vi "Init.vi"(8 "error in (no error)":errorcluster, 11 "Data in":refnum<class "Blackboard_Boolean.lvclass">) -> (0 "error out":errorcluster, 3 "Data out":refnum<class "Blackboard_Boolean.lvclass">)   [LabVIEW 2021, in "Blackboard_Boolean.lvclass"]
doc: "Abstract Data Classes 2.1.1.12\nTim Streeter - TSA\nCopyright (c) 2024, TSA"
uses:
  Blackboard_Boolean.lvclass
  Blackboard_Boolean.lvclass/Blackboard_Boolean.ctl
  Blackboard.lvclass
  <vilib>/TSA/Abstract Data Classes/Abs_Types/Type/Abs_Type.lvclass
  <vilib>/Utility/Data Type/Type Definitions/Data Type.ctl
  <vilib>/Utility/Data Type/NI_Data Type.lvlib
  C:/Program Files (x86)/National Instruments/LabVIEW 2021/vi.lib/TSA/Abstract Data Classes/Abs_Types/Boolean/Abs_Boolean.lvclass
  C:/Program Files (x86)/National Instruments/LabVIEW 2021/vi.lib/TSA/Abstract Data Classes/Abs_Types/Value/Abs_Value.lvclass
  C:/Program Files (x86)/National Instruments/LabVIEW 2021/vi.lib/TSA/Abstract Data Classes/Abs_Types/Type/Abs_Type.lvclass
  C:/Users/Tim/Documents/GitHub/LV_Behaviour_Tree/Source/Blackboard/Support/Bool/Blackboard_Boolean.lvclass
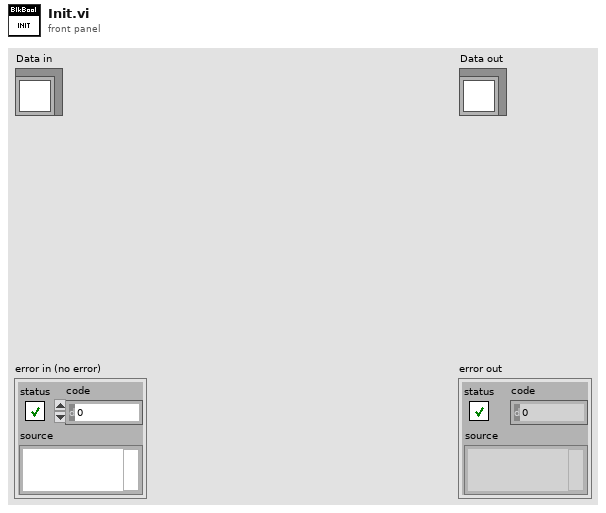
[diagram p1: front panel]
types:
  T1 = typedef "NI_Data Type.lvlib/Data Type.ctl" = enum8{"Invalid Type", "Void", "I8", "I16", "I32", "I64", "U8", "U16", "U32", "U64", "Single Float", "Double Float", "Extended Float", "Single Complex", "Double Complex", "Extended Complex", "Enum U8", "Enum U16", "Enum U32", "Enum U64", "Single Float With Unit", "Double Float With Unit", "Extended Float With Unit", "Single Complex with Unit", "Double Complex with Unit", "Extended Complex with Unit", "Boolean", "String", "Path", "Picture", "Tag", "Array", "Cluster", "Variant", "LV Variant", "Waveform", "Timestamp", "Digital Waveform", "Digital Data", "ExpressData", "Refnum", "External Data", "VI", "Poly VI", "LabVIEW Class Instance", "Fixed Point", "Set Collection", "Map Collection"}
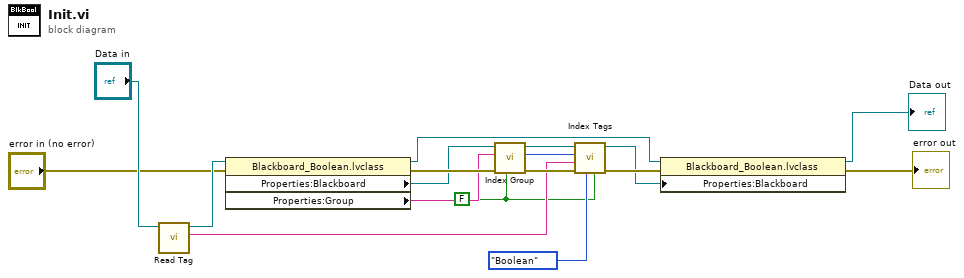
[diagram p0: block diagram]
diagram:
  w1 = FALSE ("Don't Create")
  n1 = call <vilib>:"Read Tag.vi"("Abs_Type in"="Data in") -> ("Tag"=w12:string, "Abs_Type out"=w14:refnum<class "Blackboard_Boolean.lvclass">)  [unwired: 9 in]
  n2 = property class="Blackboard_Boolean.lvclass"(reference=w14, error in="error in (no error)") -> (reference out=w3:refnum<class "Blackboard_Boolean.lvclass">, error out=w16:errorcluster, "Properties:Blackboard"=w10:refnum<class "Blackboard.lvclass">, "Properties:Group"=w9:string)
  n3 = call "Index Group.vi"("Don't Create"=w1, "error in (no error)"=w16, "Group"=w9, "bt_Blackboard in"=w10) -> ("error out"=w15:errorcluster, "Index"=w6:i32, "bt_Blackboard out"=w17:refnum<class "Blackboard.lvclass">)  [unwired: 5 in]
  n4 = call "Index Tags.vi"("Don't Create"=w1, "Tag Type"=Data_Type."Boolean", "error in (no error)"=w15, "Tag"=w12, "Group Index"=w6, "bt_Blackboard in"=w17) -> ("error out"=w8:errorcluster, "bt_Blackboard out"=w7:refnum<class "Blackboard.lvclass">)  [unwired: 2 in, 2 out]
  n5 = property class="Blackboard_Boolean.lvclass"(reference=w3, error in=w8, "Properties:Blackboard"=w7) -> (reference out=→"Data out":refnum<class "Blackboard_Boolean.lvclass">, error out=→"error out":errorcluster)
